vi "CF_Z_Bridge_to_DSC.vi"(8 "error in (no error)":errorcluster, 9 "calibration string":string="CMN 187_TC_2-29, 140701_OuterSP (fit from fit, self defined fx)_TC, 140702_Solenoid (Right, fit from fit, self defined fx)_TC, RuO2_10K_TC, RuO2_10K_TC, No Calibration, No Calibration, No Calibration, No Calibration, No Calibration", 10 "description string":string="3K, Still, 50 mK, MC, MC, , , , , ", 11 "dbl":dbl[](array[numeric])=[-1e+30, 3977.4776241280374, 3649.809852131724, 0.0, 17313.58847758918, 0.0, 0.0, 0.0, 0.0, 0.0, -5.724e-36, 4025.436136585684, 4054.3239935153424, nan, 4258.3107502810735, 0.0, 0.0, 0.0, 0.0, 0.0]) -> (0 "error out":errorcluster)   [LabVIEW 2013]
panel:
  in  "calibration string var":refnum<k21>="ni.var.psp://housesoftheholy/Leiden CF900/CF_TC_Z_calibration"
  in  "description string var":refnum<k21>="ni.var.psp://housesoftheholy/Leiden CF900/CF_TC_Z_description"
  in  "dbl var":refnum<k21>[](array[refnum])=["ni.var.psp://housesoftheholy/Leiden CF900/CF_TC_Z_R0", "ni.var.psp://housesoftheholy/Leiden CF900/CF_TC_Z_R1", "ni.var.psp://housesoftheholy/Leiden CF900/CF_TC_Z_R2", "ni.var.psp://housesoftheholy/Leiden CF900/CF_TC_Z_R3", "ni.var.psp://housesoftheholy/Leiden CF900/CF_TC_Z_R4", "ni.var.psp://housesoftheholy/Leiden CF900/CF_TC_Z_R5", "ni.var.psp://housesoftheholy/Leiden CF900/CF_TC_Z_R6", "ni.var.psp://housesoftheholy/Leiden CF900/CF_TC_Z_R7", "ni.var.psp://housesoftheholy/Leiden CF900/CF_TC_Z_R8", "ni.var.psp://housesoftheholy/Leiden CF900/CF_TC_Z_R9", "ni.var.psp://housesoftheholy/Leiden CF900/CF_TC_Z_T0", "ni.var.psp://housesoftheholy/Leiden CF900/CF_TC_Z_T1", "ni.var.psp://housesoftheholy/Leiden CF900/CF_TC_Z_T2", "ni.var.psp://housesoftheholy/Leiden CF900/CF_TC_Z_T3", "ni.var.psp://housesoftheholy/Leiden CF900/CF_TC_Z_T4", "ni.var.psp://housesoftheholy/Leiden CF900/CF_TC_Z_T5", "ni.var.psp://housesoftheholy/Leiden CF900/CF_TC_Z_T6", "ni.var.psp://housesoftheholy/Leiden CF900/CF_TC_Z_T7", "ni.var.psp://housesoftheholy/Leiden CF900/CF_TC_Z_T8", "ni.var.psp://housesoftheholy/Leiden CF900/CF_TC_Z_T9"]
  # "CF Impedence Bridge to DSC"
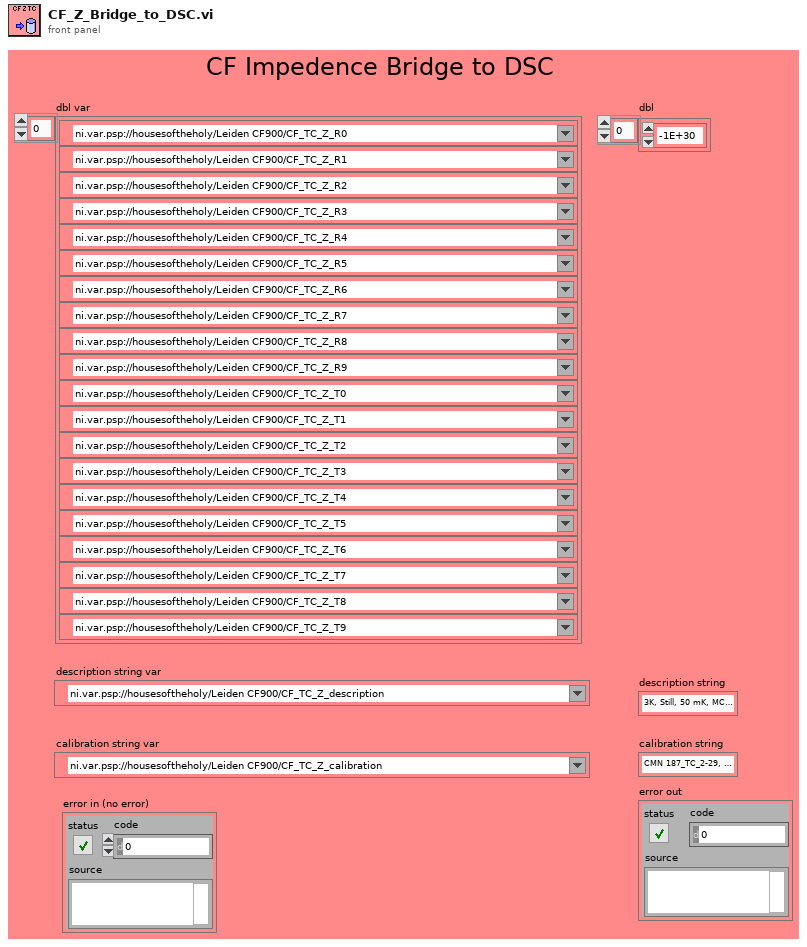
[diagram p1: front panel]
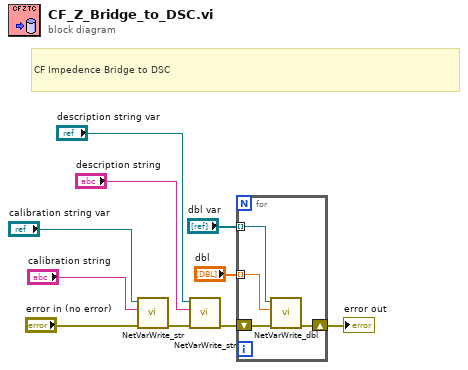
[diagram p0: block diagram]
diagram:
  # "CF Impedence Bridge to DSC"
  n1 = call "NetVarWrite_str.vi"("error in (no error)"="error in (no error)", "String"="calibration string", "Refnum in"="calibration string var") -> ("error out"=w5:errorcluster)  [unwired: 8 in]
  n2 = call "NetVarWrite_str.vi"("error in (no error)"=w5, "String"="description string", "Refnum in"="description string var") -> ("error out"=w4:errorcluster)  [unwired: 8 in]
  n3 = for {
    tunnel: "dbl var" -> [w14] mode=indexing
    tunnel: "dbl" -> [w13] mode=indexing
    shift-right: [w11] -> w8
    shift-left: w4 -> [w12]
    n4 = call "NetVarWrite_dbl.vi"("error in (no error)"=w12, "Numeric"=w13, "Refnum in"=w14) -> ("error out"=w11:errorcluster)  [unwired: 8 in]
  }
  "error out" <- w8
